vi "TSCAN_GetSignalValue_CAN.vi"(6 "All_ID":i32[](array[numeric]) format="%x", 7 "Message":T1, 8 "错误输入（无错误）":errorcluster, 9 "ALLSignalName":string[][](array[string]), 10 "ALLMessage":string[](array[string]), 11 "路径输入":path) -> (0 "错误输出":errorcluster, 1 "SigValue":dbl[](array[numeric]), 2 "SigName":string[](array[string]), 3 "路径输出":path, 4 "Message Name":string[](array[string]))   [LabVIEW 2014]
panel:
  out "Element index":i32
  out "tsdb_load_can_db":i32
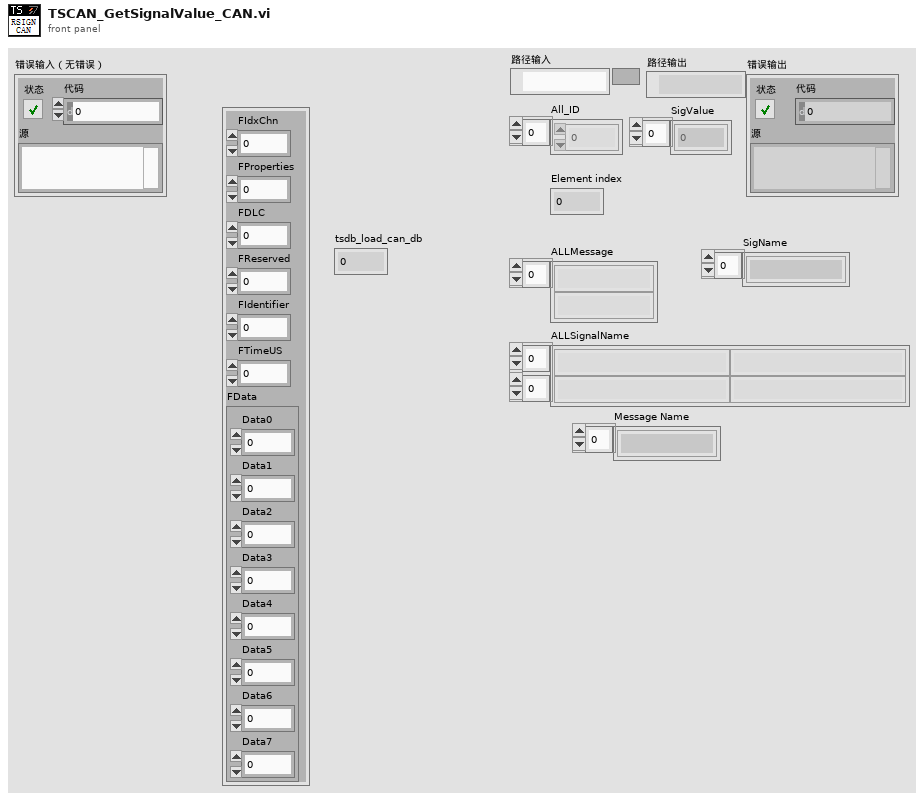
[diagram p1: front panel]
types:
  T1 = cluster{"FIdxChn":u8, "FProperties":u8, "FDLC":u8, "FReserved":u8, "FIdentifier":i32, "FTimeUS":u64, "FData":cluster{"Data0":u8, "Data1":u8, "Data2":u8, "Data3":u8, "Data4":u8, "Data5":u8, "Data6":u8, "Data7":u8}}
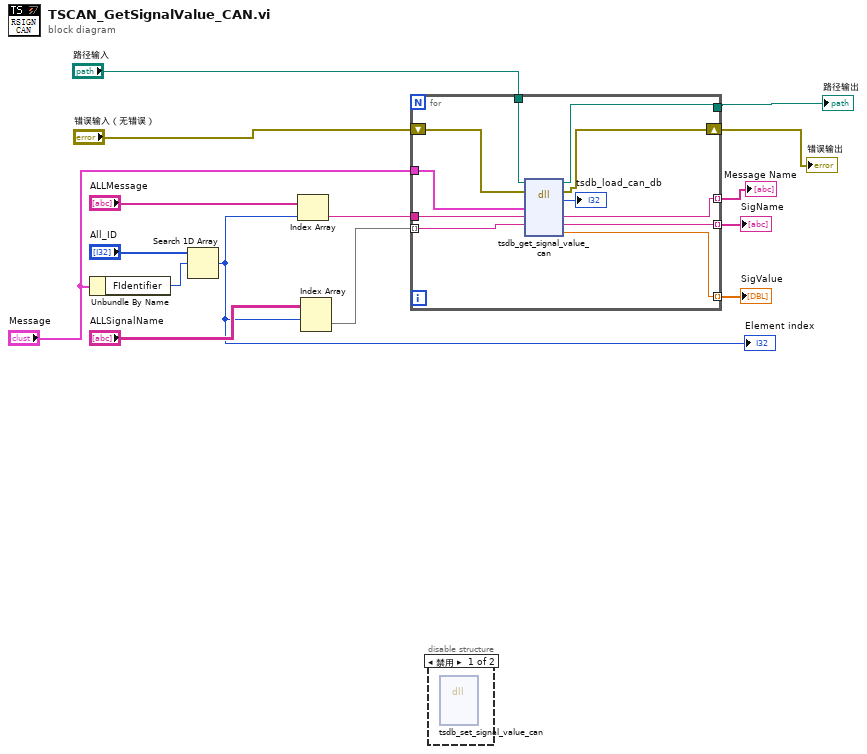
[diagram p0: block diagram]
diagram:
  n1 = Unbundle By Name("Message") -> ("FIdentifier"=w13:i32)
  n2 = Search 1D Array(1D array="All_ID", element=w13) -> (index of element=w9:i32)  [unwired: 1 in]
  "Element index" <- w9
  n3 = Index Array(array="ALLMessage", index=w9) -> (element=w11:string)
  n4 = Index Array(array="ALLSignalName", index (row)=w9) -> (element=w8:string[])  [unwired: 1 in]
  n5 = for {
    tunnel: "Message" -> [w26]
    tunnel: w11 -> [w25]
    tunnel: w8 -> [w23] mode=indexing
    tunnel: [w22] -> w7 mode=indexing
    tunnel: [w21] -> w6 mode=indexing
    tunnel: "路径输入" -> [w18]
    tunnel: [w17] -> w2
    shift-right: [w19] -> w4
    shift-left: "错误输入（无错误）" -> [w20]
    tunnel: [w16] -> w1 mode=indexing
    n6 = dll-call lib="PTH27abs EDemo同星\nTSCAN_V1.0ConfigTSMaster.dll" fn="tsdb_get_signal_value_can"(path in=w18, error in=w20, "CANObJ"=w26, "Message"=w25, "Signal"=w23) -> (path out=w17:path, error out=w19:errorcluster, "tsdb_get_signal_value_can"=→"tsdb_load_can_db":i32, "Message"=w16:string, "Signal"=w21:string, "SigValue"=w22:dbl)  [unwired: 3 in]
  }
  "SigValue" <- w7
  "SigName" <- w6
  "错误输出" <- w4
  "路径输出" <- w2
  "Message Name" <- w1
  n7 = disable-structure shown="禁用" {
    frame Disabled {
      n8 = dll-call lib="PTH27abs EDemo同星\nTSCAN_V1.0ConfigTSMaster.dll" fn="tsdb_set_signal_value_can"() -> ()  [unwired: 10 in, 2 out]
    }
    frame Enabled {
    }
  }
